vi "Pressure_statistic with temperature(multiple regime).vi"() -> ()   [LabVIEW 2014]
uses:
  <vilib>/Utility/error.llb/DialogType.ctl
  Instance          11 26Saved   Pressure_statistic .vi
  Instance           1 26Saved   Pressure_statistic .vi
  Instance           7 26Saved   Pressure_statistic .vi
  Instance           6 26Saved   Pressure_statistic .vi
  Instance          18 26Saved   Pressure_statistic .vi
  Instance           2 26Saved   Pressure_statistic .vi
  Instance           5 26Saved   Pressure_statistic .vi
  <vilib>/Utility/file.llb/Write To Spreadsheet File (DBL).vi
  Instance           4 26Saved   Pressure_statistic .vi
  Instance           9 26Saved   Pressure_statistic .vi
  Instance           8 26Saved   Pressure_statistic .vi
  <instrlib>/Fluke 884X Series/Public/Data/Read (Multiple Points).vi
  Instance          17 26Saved   Pressure_statistic .vi
  Instance          16 26Saved   Pressure_statistic .vi
  <instrlib>/Fluke 884X Series/Fluke 884X Series.lvlib
panel:
  in  "mkv per degree(thermocouple type)":dbl
  out "T,C":dbl
  out "T,K":dbl
  in  "Tkomn, C":dbl
  in  "Timeout":i32=10000
  in  "Sample Count (10)":i32=10
  in  "Manual Range (1.0)":dbl=1.0
  in  "Auto Range (T:Enable)":bool=TRUE
  in  "Function (0: DC Voltage)":u16(ring) items=["DC Voltage", "AC Voltage", "2 - Wire Resistance", "4 - Wire Resistance", "DC Current", "AC Current", "Frequency", "Period", "Continuity", "Diode Checking", "Temperature", "Capacitance"]
  in  "Manual Resolution (5.5 Digits)":dbl(ring)=5.5 items=["4.5"=4.5, "5.5"=5.5, "6.5"=6.5]
  out "Temperature":dbl
  out "Temperature from Fluke884X":dbl[](graph)
  in  "VISA resource name":refnum<visa-resource-name>
  in  "Serial Configuration":T1={"Baud Rate"=9600, "Parity"=0, "Data Bits"=8, "Stop Bits"=10, "Flow Control"=0} {"Flow Control" items=["None", "XON/XOFF", "RTS/CTS", "XON/XOFF & RTS/CTS", "DTR/DSR", "XON/XOFF & DTR/DSR"]; "Stop Bits" items=["1.0"=10, "1.5"=15, "2.0"=20]; "Data Bits" items=["7"=7, "8"=8]; "Parity" items=["None", "Odd", "Even", "Mark", "Space"]; "Baud Rate" items=["300"=300, "600"=600, "1200"=1200, "2400"=2400, "4800"=4800, "9600"=9600, "19200"=19200]}
  in  "Filter 2":bool
  in  "Case Constant\n(See Context Help)":bool=TRUE
  in  "Write":bool
  out "P, V":dbl[](array[numeric])
  out "Waveform Graph 2":dynamicdata(graph)
  out "Waveform Graph":dynamicdata(graph)
  in  "Fourier transform":bool
  out "Pressure Frequency":dbl
  out "Pressure Amplitude":dbl
  in  "Filter":bool
  in  "Fourier transform":bool
  out "Responce Frequency":dbl
  out "Responce Amplitude":dbl
  in  "Write to file":bool
  in  "stop":bool
  # "Responce"
  # "Pressure"
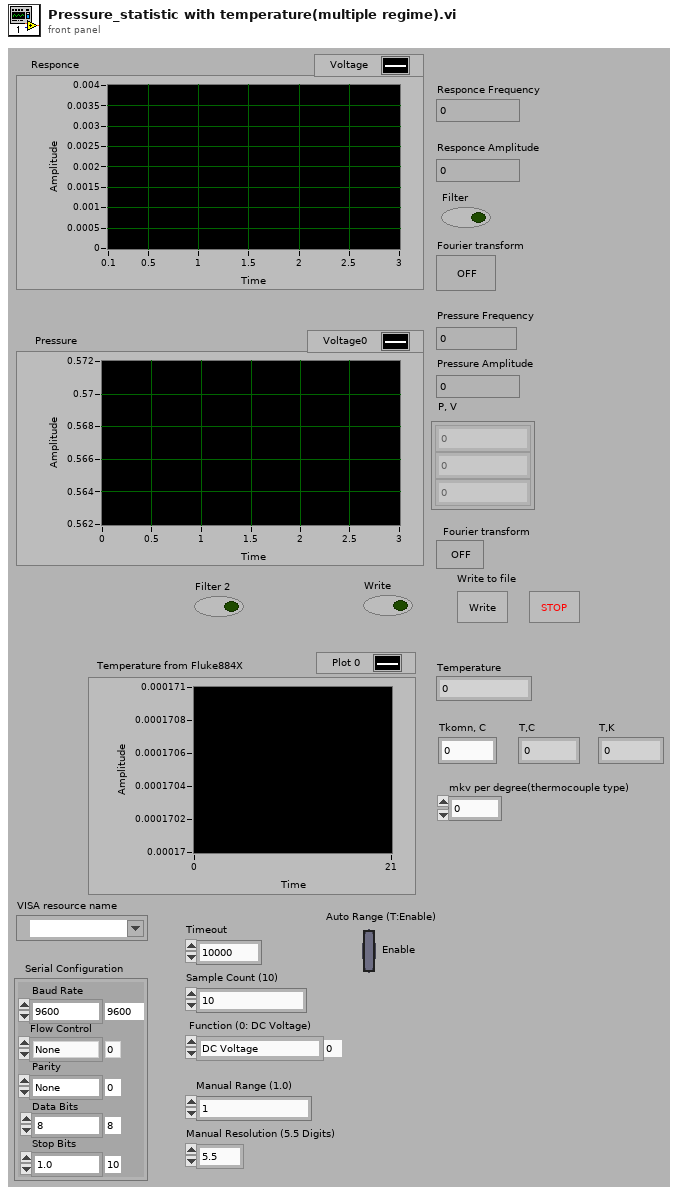
[diagram p1: front panel]
types:
  T1 = cluster{"Baud Rate":u32, "Parity":u16, "Data Bits":u16, "Stop Bits":u16, "Flow Control":u16}
  T2 = typedef "DialogType.ctl" = u16
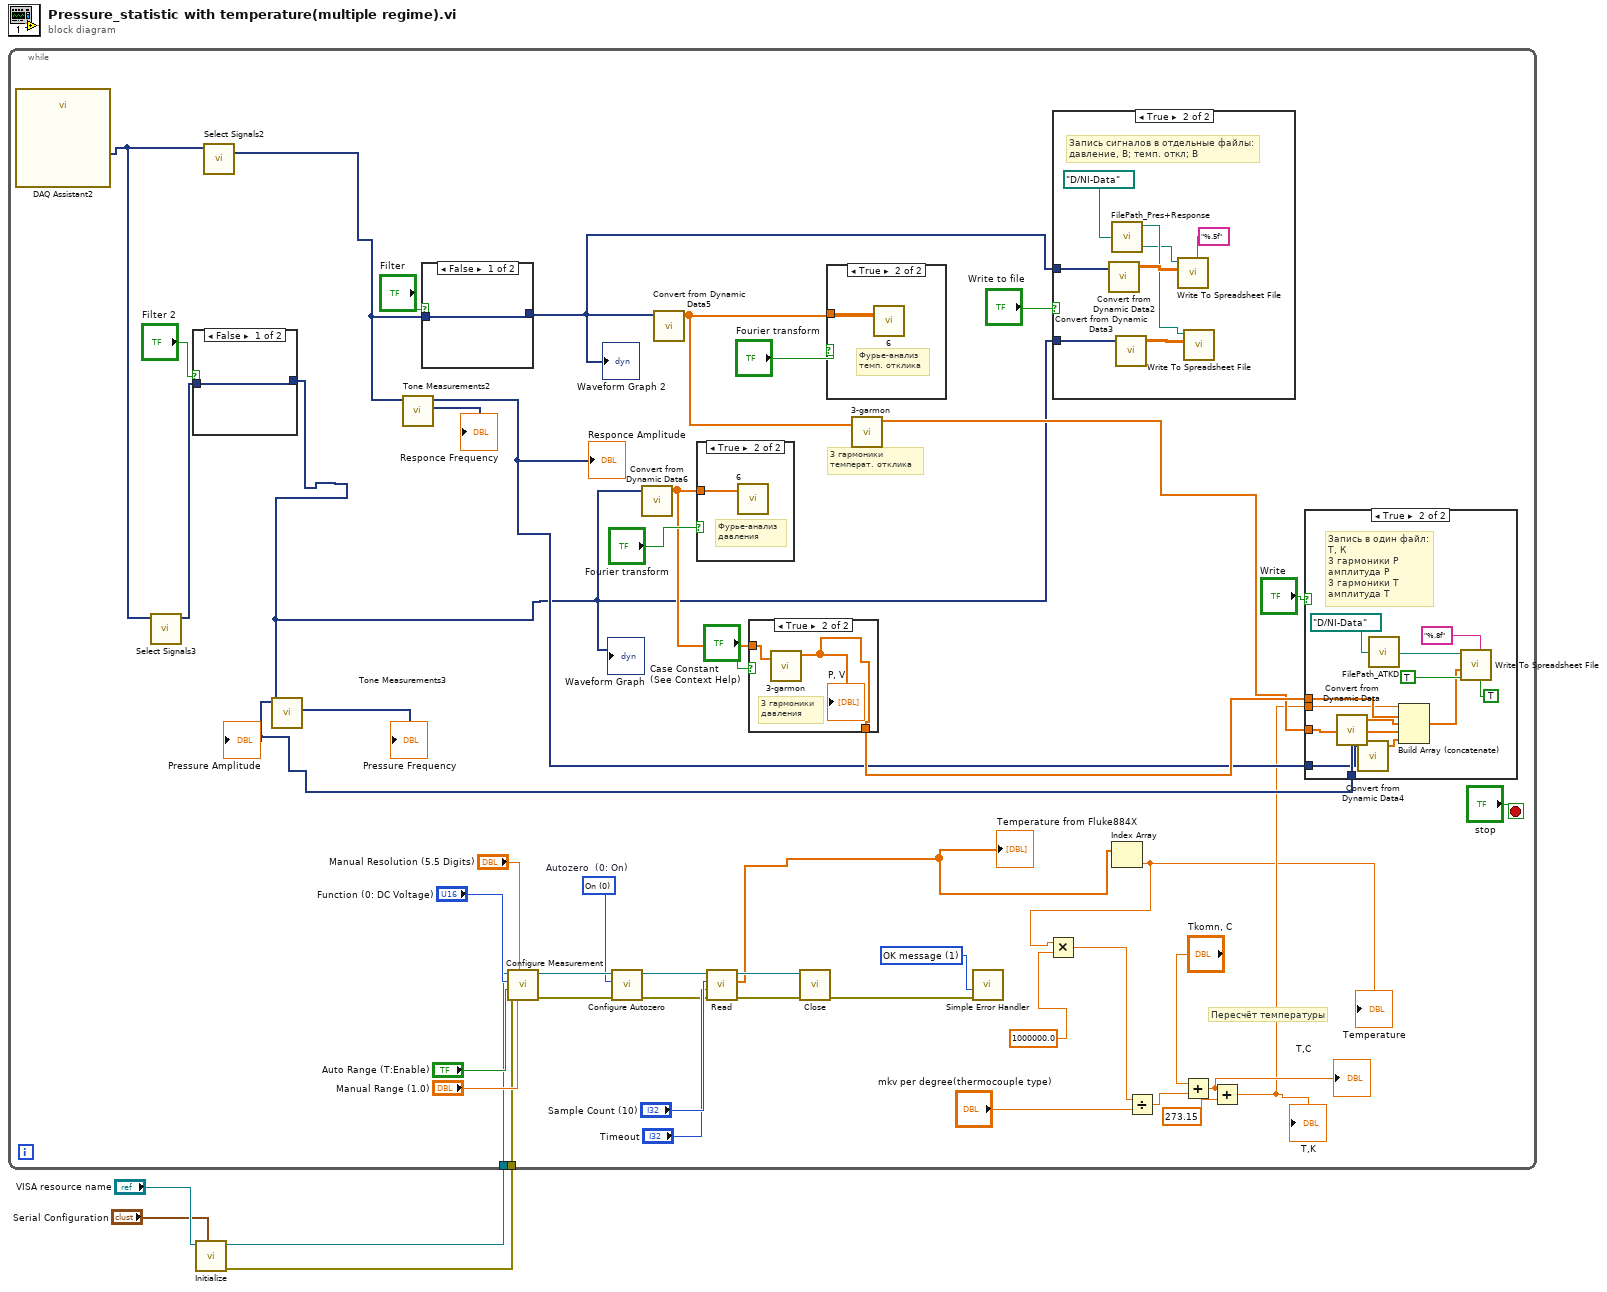
[diagram p0: block diagram]
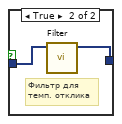
[diagram p2: hidden frame]
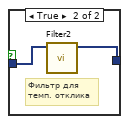
[diagram p6: hidden frame]
diagram:
  n1 = call <instrlib>:"Initialize.vi"("Serial Configuration"="Serial Configuration", "VISA resource name"="VISA resource name") -> ("error out"=w3:errorcluster, "VISA resource name out"=w4:refnum<visa-resource-name>)  [unwired: 8 in]
  n2 = while {
    tunnel: w4 -> [w16]
    tunnel: w3 -> [w15]
    stop <- "stop" stop-if-true
    w17 = u16 0 items=["On", "Off", "Once"]  # Autozero  (0: On)
    w31 = T2 1 items=["no dialog", "OK message", "continue or stop message", "OK message + warnings", "continue/stop + warnings"] ("type of dialog (OK msg:1)")
    # "Пересчёт температуры"
    # "3 гармоники\nтемперат. отклика"
    n3 = call "DAQ Assistant2"() -> ("data"=w43:dynamicdata)  [unwired: 2 in, 9 out]
    n4 = call "Select Signals3"("Signals"=w43) -> ("Signal Out"=w34:dynamicdata)  [unwired: 1 in, 9 out]
    n5 = case shown="False" "Filter 2" {
      tunnel: w34 -> [w53 w55]
      tunnel: [w53 w54] -> w32
      frame False {
      }
      frame True {
        # "Фильтр для\nтемп. отклика"
        n6 = call "Filter"("Signal"=w55) -> ("Filtered Signal"=w54:dynamicdata)  [unwired: 2 in, 8 out]
      }
    }
    "Waveform Graph" <- w32
    n7 = call "Select Signals2"("Signals"=w43) -> ("Signal Out"=w47:dynamicdata)  [unwired: 1 in, 9 out]
    n8 = call "Tone Measurements3"("Signals"=w32) -> ("Frequency"=→"Pressure Frequency":dynamicdata, "Amplitude"=w36:dynamicdata)  [unwired: 1 in, 8 out]
    "Pressure Amplitude" <- w36
    n9 = call "Tone Measurements2"("Signals"=w47) -> ("Frequency"=→"Responce Frequency":dynamicdata, "Amplitude"=w35:dynamicdata)  [unwired: 1 in, 8 out]
    "Responce Amplitude" <- w35
    n10 = case shown="False" "Filter" {
      tunnel: w47 -> [w72 w74]
      tunnel: [w72 w73] -> w44
      frame False {
      }
      frame True {
        # "Фильтр для\nтемп. отклика"
        n11 = call "Filter2"("Signal"=w74) -> ("Filtered Signal"=w73:dynamicdata)  [unwired: 2 in, 8 out]
      }
    }
    "Waveform Graph 2" <- w44
    n12 = call <instrlib>:"Configure Measurement.vi"("Manual Range (1.0)"="Manual Range (1.0)", "Manual Resolution (5.5 Digits)"="Manual Resolution (5.5 Digits)", "error in (no error)"=w15, "Auto Range (T:Enable)"="Auto Range (T:Enable)", "Function (0: DC Voltage)"="Function (0: DC Voltage)", "VISA resource name"=w16) -> ("error out"=w21:errorcluster, "VISA resource name out"=w20:refnum<visa-resource-name>)  [unwired: 4 in]
    n13 = call <instrlib>:"Configure Autozero.vi"("error in (no error)"=w21, "Autozero  (0: On)"=w17, "VISA resource name"=w20) -> ("error out"=w18:errorcluster, "VISA resource name out"=w19:refnum<visa-resource-name>)  [unwired: 7 in]
    n14 = call "Convert from Dynamic Data6"("Dynamic Data Type"=w32) -> ("Array"=w39:dbl[])  [unwired: 3 out]
    n15 = call "Convert from Dynamic Data5"("Dynamic Data Type"=w44) -> ("Array"=w42:dbl[])  [unwired: 3 out]
    n16 = case shown="True" "Fourier transform" {
      tunnel: w39 -> [_ w71]
      frame False {
      }
      frame True {
        # "Фурье-анализ\nдавления"
        n17 = call "6.vi"("X"=w71) -> ()  [unwired: 7 out]
      }
    }
    n18 = call-poly <instrlib>:"Read.vi"("error in (no error)"=w18, "Timeout (10000 ms)"="Timeout", "Sample Count (1)"="Sample Count (10)", "VISA resource name"=w19) -> ("error out"=w28:errorcluster, "Measurements"=w10:dbl[], "VISA resource name out"=w29:refnum<visa-resource-name>)  [unwired: 5 in]
    "Temperature from Fluke884X" <- w10
    n19 = case shown="True" "Case Constant\n(See Context Help)" {
      tunnel: w39 -> [_ w70]
      tunnel: [_ w69] -> w38
      frame False {
      }
      frame True {
        # "3 гармоники\nдавления"
        n20 = call "3-garmon.vi"("X"=w70) -> ("A"=w69:dbl[])  [unwired: 6 out]
        "P, V" <- w69
      }
    }
    n21 = call <instrlib>:"Close.vi"("error in (no error)"=w28, "VISA resource name"=w29) -> ("error out"=w30:errorcluster)  [unwired: 9 in]
    n22 = case shown="True" "Fourier transform" {
      tunnel: w42 -> [_ w75]
      frame False {
      }
      frame True {
        # "Фурье-анализ\nтемп. отклика"
        n23 = call "6.vi"("X"=w75) -> ()  [unwired: 7 out]
      }
    }
    n24 = call "3-garmon.vi"("X"=w42) -> ("A"=w37:dbl[])  [unwired: 6 out]
    n25 = call <vilib>:"Simple Error Handler.vi"("type of dialog (OK msg:1)"=w31, "error in (no error)"=w30) -> ()  [unwired: 3 in, 5 out]
    n26 = case shown="True" "Write to file" {
      tunnel: w44 -> [_ w83]
      tunnel: w32 -> [_ w80]
      frame False {
      }
      frame True {
        # "Запись сигналов в отдельные файлы:\nдавление, В; темп. откл; В"
        n27 = call "Convert from Dynamic Data2"("Dynamic Data Type"=w83) -> ("Array"=w82:dbl[][])  [unwired: 3 out]
        n28 = call "FilePath_Pres+Response.vi"("base folder path"=path "D:/NI-Data") -> ("Pressure"=w78:path, "Response"=w77:path)  [unwired: 1 out]
        n29 = call "Convert from Dynamic Data3"("Dynamic Data Type"=w80) -> ("Array"=w81:dbl[][])  [unwired: 3 out]
        n30 = call-poly <vilib>:"Write To Spreadsheet File.vi"("format (%.3f)"="%.5f", "2D data"=w82, "file path (dialog if empty)"=w77) -> ()  [unwired: 3 in, 3 out]
        n31 = call-poly <vilib>:"Write To Spreadsheet File.vi"("2D data"=w81, "file path (dialog if empty)"=w78) -> ()  [unwired: 4 in, 3 out]
      }
    }
    n32 = Index Array(array=w10) -> (element=w7:dbl)  [unwired: 1 in]
    "Temperature" <- w7
    n33 = Multiply(x=w7, y=1000000.0) -> (x*y=w5:dbl)
    n34 = Divide(x=w5, y="mkv per degree(thermocouple type)") -> (x/y=w13:dbl)
    n35 = Add(x="Tkomn, C", y=w13) -> (x+y=w11:dbl)
    "T,C" <- w11
    n36 = Add(x=w11, y=273.15) -> (x+y=w8:dbl)
    "T,K" <- w8
    n37 = case shown="True" "Write" {
      tunnel: w38 -> [_ w68]
      tunnel: w37 -> [_ w62]
      tunnel: w36 -> [_ w61]
      tunnel: w35 -> [_ w59]
      tunnel: w8 -> [_ w56]
      frame False {
      }
      frame True {
        # "Запись в один файл:\nТ, К\n3 гармоники P\nамплитуда P\n3 гармоники Т\nамплитуда Т"
        n38 = call "Convert from Dynamic Data"("Dynamic Data Type"=w61) -> ("Array"=w60:dbl[])  [unwired: 3 out]
        n39 = call "Convert from Dynamic Data4"("Dynamic Data Type"=w59) -> ("Array"=w58:dbl[])  [unwired: 3 out]
        n40 = call "FilePath_ATKD.vi"("base folder path"=path "D:/NI-Data") -> ("ATKD"=w67:path)  [unwired: 3 out]
        n41 = Build Array (concatenate)(w56, w68, w60, w62, w58) -> (w57:dbl[])
        n42 = call-poly <vilib>:"Write To Spreadsheet File.vi"("transpose? (no:F)"=TRUE, "format (%.3f)"="%.8f", "append to file? (new file:F)"=TRUE, "1D data"=w57, "file path (dialog if empty)"=w67) -> ()  [unwired: 1 in, 3 out]
      }
    }
  }
